vi "Load Waveform Data.vi"(4 "error in":errorcluster, 5 "# Records (1)":i32=1, 6 "# Records to Skip (0)":i32, 7 "Source File":path) -> (0 "error out":errorcluster, 3 "Data":waveform(dbl)[][](array[waveform]))   [LabVIEW 2013]
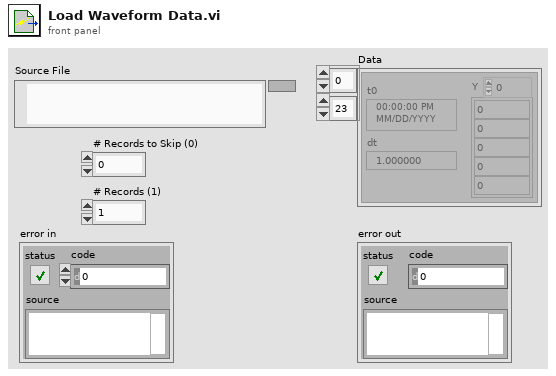
[diagram p1: front panel]
types:
  T1 = enum16{"big-endian, network order", "native, host order", "little-endian"}
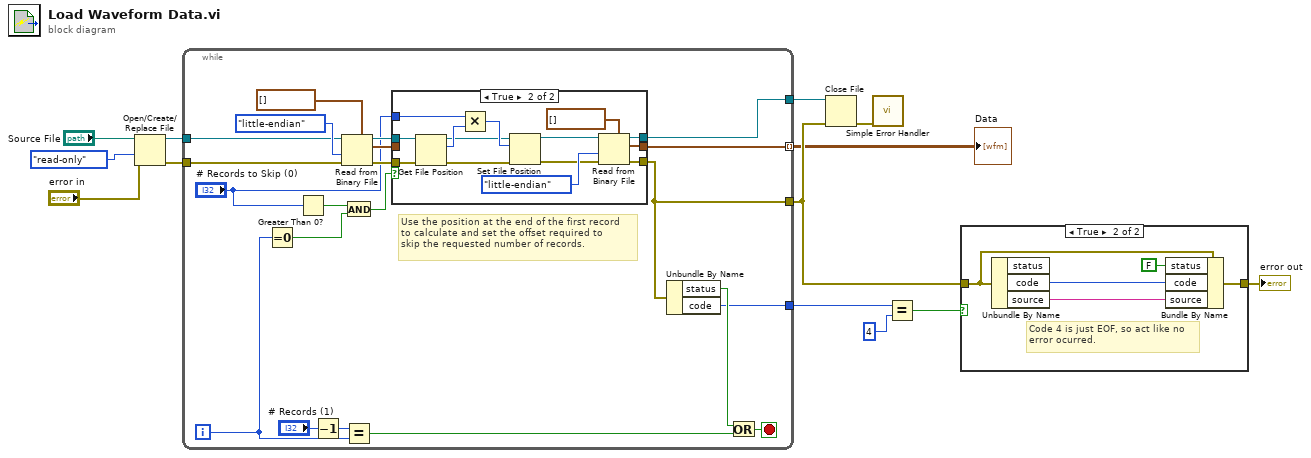
[diagram p0: block diagram]
diagram:
  n1 = Open/Create/Replace File(file path (use dialog)="Source File", error in="error in", access (0:read/write)=enum16{"read/write", "read-only", "write-only"}."read-only") -> (refnum out=w10:refnum<file>, error out=w9:errorcluster)  [unwired: 3 in, 1 out]
  n2 = while {
    tunnel: [w19] -> w2 mode=indexing
    tunnel: [w31] -> w6
    tunnel: w10 -> [w28]
    tunnel: w9 -> [w27]
    tunnel: [w17] -> w4
    tunnel: [w18] -> w3
    i -> [w26]
    stop <- w34 stop-if-true
    # "Use the position at the end of the first record\nto calculate and set the offset required to\nskip the requested number of records."
    n3 = Equal To 0?(x=w26) -> (x = 0?=w21:bool)
    n4 = Greater Than 0?(x="# Records to Skip (0)") -> (x > 0?=w22:bool)
    n5 = Decrement(x="# Records (1)") -> (x-1=w15:i32)
    n6 = Read from Binary File(5:waveform(dbl)[] [] ("Difference"), 8:w27, 9:T1."little-endian" ("byte order (0:big-endian, network order)"), 11:w28) -> (0:w24:errorcluster, 2:w20:waveform(dbl)[], 3:w25:refnum<file>)  [unwired: 2 in, 1 out]
    n7 = And(x=w22, y=w21) -> (x .and. y?=w23:bool)
    n8 = Equal?(x=w15, y=w26) -> (x = y?=w32:bool)
    n9 = case shown="True" w23 {
      tunnel: w25 -> [w36 w51]
      tunnel: w24 -> [w35 w50]
      tunnel: "# Records to Skip (0)" -> [_ w48]
      tunnel: w20 -> [w37 _]
      tunnel: [w37 w40] -> w19
      tunnel: [w35 w39] -> w17
      tunnel: [w36 w38] -> w18
      frame False {
      }
      frame True {
        n10 = Get File Position(4:w50, 7:w51) -> (0:w46:errorcluster, 2:w49:i64, 3:w45:refnum<file>)
        n11 = Multiply(x=w48, y=w49) -> (x*y=w47:i64)
        n12 = Set File Position(offset (in bytes) (0)=w47, refnum=w45, error in=w46) -> (refnum out=w43:refnum<file>, error out=w41:errorcluster)  [unwired: 1 in]
        n13 = Read from Binary File(5:waveform(dbl)[] [] ("Difference"), 8:w41, 9:T1."little-endian" ("byte order (0:big-endian, network order)"), 11:w43) -> (0:w39:errorcluster, 2:w40:waveform(dbl)[], 3:w38:refnum<file>)  [unwired: 2 in, 1 out]
      }
    }
    n14 = Unbundle By Name(w17) -> ("status"=w33:bool, "code"=w31:i32)
    n15 = Or(x=w33, y=w32) -> (x .or. y?=w34:bool)
  }
  "Data" <- w2
  n16 = Close File(refnum=w3, error in=w4) -> (error out=w1:errorcluster)  [unwired: 1 out]
  n17 = call <vilib>:"Simple Error Handler.vi"("error in (no error)"=w1) -> ()  [unwired: 4 in, 5 out]
  n18 = Equal?(x=w6, y=4 ("code")) -> (x = y?=w8:bool)
  n19 = case shown="True" w8 {
    tunnel: w4 -> [w52 w57]
    tunnel: [w52 w53] -> w5
    frame False {
    }
    frame True {
      # "Code 4 is just EOF, so act like no\nerror ocurred."
      n20 = Unbundle By Name(w57) -> ("code"=w56:i32, "source"=w55:string)  [unwired: 1 out]
      n21 = Bundle By Name(cluster=w57, "status"=FALSE, "code"=w56, "source"=w55) -> (w53:errorcluster)
    }
  }
  "error out" <- w5
